vi "Filter.vi"(8 "error in (no error)":errorcluster, 11 "_Msg-Filter in":refnum<class "_Msg-Filter.lvclass">) -> (0 "error out":errorcluster, 2 "Found?":bool)   [LabVIEW 2020, in "MailboxClient.lvlib" / "_Msg-Filter.lvclass"]
uses:
  _Msg-Filter.lvclass
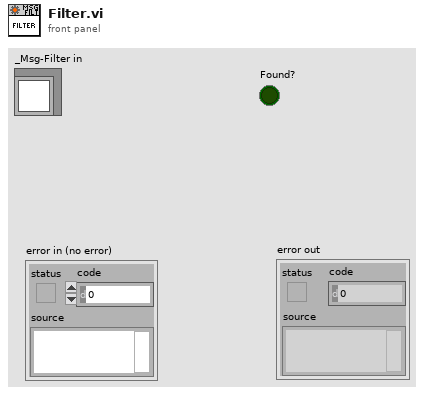
[diagram p1: front panel]
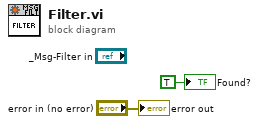
[diagram p0: block diagram]
diagram:
  "error out" <- "error in (no error)"
  "Found?" <- TRUE ("Found?")
